vi "Get Project Members.vi"(8 "error in (no error)":errorcluster, 10 "Project GID":string, 11 "Asana in":refnum<class "Asana.lvclass">) -> (0 "error out":errorcluster, 2 "data":T1(array[cluster]), 3 "Asana out":refnum<class "Asana.lvclass">)   [LabVIEW 2016, in "Asana.lvclass"]
uses:
  Asana.lvclass
  Asana.lvclass/Asana.ctl
  <vilib>/addons/_JKI.lib/REST Client/classes/REST Client/REST Client.lvclass
  <vilib>/addons/_JKI.lib/Serialization/JSON/JKI JSON Serialization.lvlib
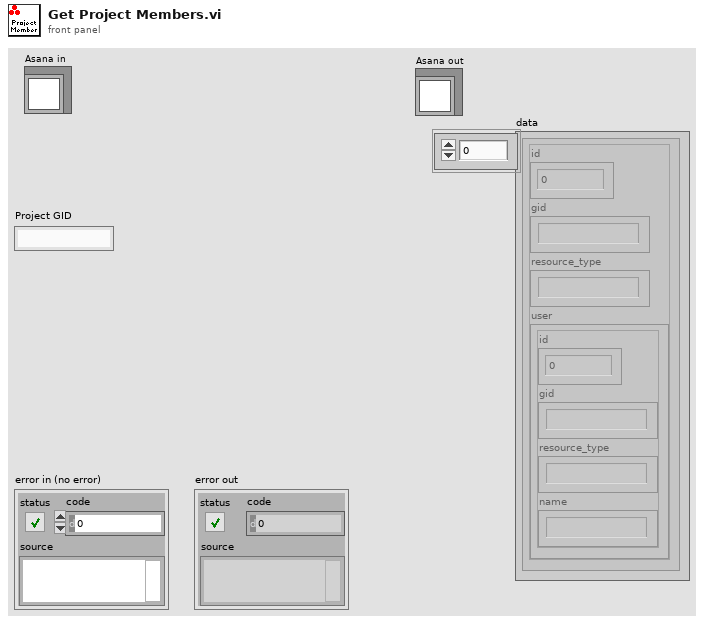
[diagram p1: front panel]
types:
  T1 = cluster{"id":i32, "gid":string, "resource_type":string, "user":cluster{"id":i32, "gid":string, "resource_type":string, "name":string}}[]
  T2 = typedef "REST Client.lvlib/REST Client.lvclass/HTTP Header.ctl" = cluster{"header":string, "value":string}
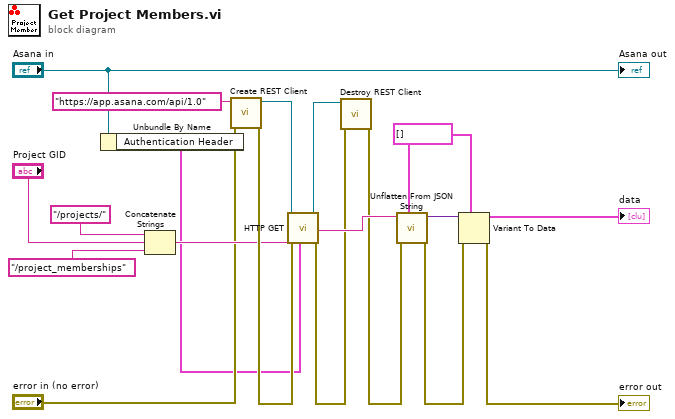
[diagram p0: block diagram]
diagram:
  w6 = T1 []
  n1 = Unbundle By Name("Asana in") -> ("Authentication Header"=w3:T2[])
  n2 = Concatenate Strings("/projects/" ("string"), "Project GID", "/project_memberships" ("string")) -> (w14:string)
  n3 = call <vilib>:"Create REST Client.vi"("error in (no error)"="error in (no error)", "Base URL"="https://app.asana.com/api/1.0") -> ("error out"=w17:errorcluster, "REST Client out"=w19:refnum<class "REST Client.lvclass">)  [unwired: 8 in]
  n4 = call-dynamic "HTTP GET.vi"("request specific headers"=w3, "error in (no error)"=w17, "Path"=w14, "REST Client in"=w19) -> ("error out"=w11:errorcluster, "Response body"=w13:string, "REST Client out"=w18:refnum<class "REST Client.lvclass">)  [unwired: 2 in, 3 out]
  n5 = call-dynamic "Destroy REST Client.vi"("error in (no error)"=w11, "REST Client in"=w18) -> ("error out"=w10:errorcluster)  [unwired: 9 in]
  n6 = call <vilib>:"Unflatten From JSON String.vi"("Type and Defaults"=w6, "error in (no error)"=w10, "JSON String"=w13) -> ("error out"=w9:errorcluster, "Variant"=w12:variant)  [unwired: 7 in]
  n7 = Variant To Data(error in=w9, type=w6, Variant=w12) -> (data=→"data":T1, error out=→"error out":errorcluster)
  "Asana out" <- "Asana in"
